vi "Fianium_Temp.vi"() -> ()   [LabVIEW 2011]
uses:
  <vilib>/Platform/TimedLoop/XDataNode/timing_clust.ctl
  <vilib>/Platform/TimedLoop/XDataNode/nitl_modes.ctl
  <vilib>/Platform/TimedLoop/XDataNode/wakeup.ctl
  <vilib>/Instr/_visa.llb/VISA Configure Serial Port (Instr).vi
  <vilib>/Platform/TimedLoop/scheduler/LVUserAPI/_suppVIs/Create_1kHz_TSource.vi
  <vilib>/Platform/TimedLoop/XDataNode/XDataNode.xnode
  <vilib>/Platform/TimedLoop/XDataNode/XDNodeRunTimeDep.lvlib
panel:
  in  "Stop":bool
  out "bytes written":u32 caption="Geschriebene Bytes"
  in  "(0xA = LF)":u8=10 caption="Abschlusszeichen\n(0xA = '\\n' = LF)" format="%.0x"
  out "bytes read":u32 caption="Gelesene Bytes"
  out "String":string
  in  "stop bits":u16(ring)=10 caption="Stoppbits" items=["1.0"=10, "1.5"=15, "2.0"=20]
  in  "flow control":u16(ring) caption="Ablaufsteuerung" items=["Keine"=0, "XON/XOFF"=1, "RTS/CTS"=2, "DTR/DSR"=4]
  in  "parity":u16(ring) caption="Parität (0: keine)" items=["Keine", "Ungerade", "Gerade", "Mark", "Space"]
  in  "data bits":u16=8 caption="Datenbits (8)" min=5 max=8 step=1
  in  "baud rate":u32=19200 caption="Baudrate (9600)"
  in  "string to write":string="t?" caption="Zu schreibender String"
  in  "VISA resource name":refnum<visa-resource-name>="COM8" caption="VISA-Ressourcenname (Schreiben)"
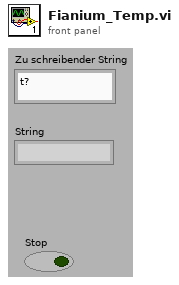
[diagram p1: front panel]
types:
  T1 = typedef "XDNodeRunTimeDep.lvlib/timing_clust.ctl" = cluster{"Expected End [f-1]":u64, "Actual End [f-1]":u64, "Finished Late? [f-1]":bool, "Expected End [i-1]":u64, "Actual End [i-1]":u64, "Finished Late? [i-1]":bool, "Expected Start [i]":u64, "Actual Start [i]":u64, "Expected Start [f]":u64, "Actual Start [f]":u64, "Source Name":string, "Structure Name":string, "Period":i64, "Deadline":i64, "Offset":i64, "Start":i64, "Priority":i32, "Timeout":i32, "Mode":T2, "Wakeup Reason":T3, "Error":errorcluster, "Source Type":string, "Secondary Source Type":string, "Global End Time":u64, "Global Start Time":u64, "Frame Duration":u64, "Iteration Duration":u64, "Assigned CPU":i32, "I/O Scan Engine Mode":u32}
  T2 = typedef "XDNodeRunTimeDep.lvlib/nitl_modes.ctl" = enum32{"No Change", "Process missed periods, maintain original phase", "Discard missed periods, maintain original phase", "Process missed periods, ignore original phase", "Discard missed periods, ignore original phase"}
  T3 = typedef "XDNodeRunTimeDep.lvlib/wakeup.ctl" = enum32{"Normal", "Aborted", "Asynchronous wakeup", "Timing source error", "Timed loop error", "Timeout"}
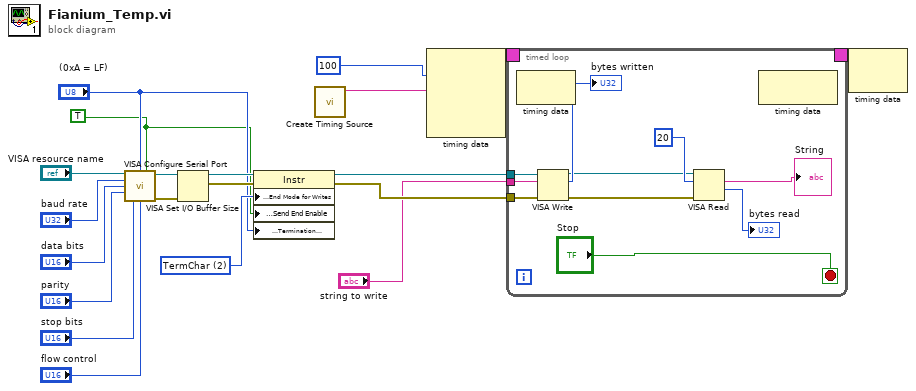
[diagram p0: block diagram]
diagram:
  w8 = TRUE
  w10 = u16 2 items=["None", "LastBit", "TermChar", "Break"] ("Serial Settings:Serial End Mode for Writes")
  n1 = call-poly "VISA Configure Serial Port"("VISA resource name"="VISA resource name", "termination char\n(0xA = '\\n' = LF)"="(0xA = LF)", "Enable Termination\nChar (T)"=w8, "baud rate (9600)"="baud rate", "data bits (8)"="data bits", "parity (0:none)"="parity", "stop bits (10: 1 bit)"="stop bits", "flow control (0:none)"="flow control") -> ("VISA resource name out"=w14:refnum<visa-resource-name>, "error out"=w13:errorcluster)  [unwired: 6 in]
  n2 = VISA Set I/O Buffer Size(VISA resource name=w14, error in (no error)=w13) -> (VISA resource name out=w11:refnum<visa-resource-name>, error out=w12:errorcluster)  [unwired: 2 in]
  n3 = property class="Instr"(reference=w11, error in=w12, "Serial Settings:End Mode for Writes"=w10, "Message Based Settings:Send End Enable"=w8, "Message Based Settings:Termination Character"="(0xA = LF)") -> (reference out=w5:refnum<visa-resource-name>, error out=w7:errorcluster)
  n4 = call-poly <vilib>:"Create Timing Source.vi"() -> ("name (out)"=w2:string)  [unwired: 10 in, 1 out]
  n5 = node-c288(100, w2) -> (w4:T1)  [unwired: 2 in]
  n6 = timed-loop {
    tunnel: w7 -> [w29]
    tunnel: "string to write" -> [w24]
    tunnel: w5 -> [w23]
    timing: w4 -> [_]
    timing-out: [_] -> w3
    stop <- "Stop" stop-if-true
    n7 = node-c288() -> ()  [unwired: 1 in, 1 out]
    n8 = VISA Write(VISA resource name=w23, write buffer=w24) -> (VISA resource name out=w22:refnum<visa-resource-name>, return count=→"bytes written":u32)  [unwired: 1 in, 1 out]
    n9 = VISA Read(VISA resource name=w22, byte count=20, error in (no error)=w29) -> (read buffer=→"String":string, return count=→"bytes read":u32)  [unwired: 2 out]
    n10 = node-c288() -> ()  [unwired: 1 in, 1 out]
  }
  n11 = node-c288(w3) -> ()  [unwired: 1 out]
